vi "File_Writing_U6Instrumentation.vi"(8 "error in (no error)":errorcluster, 10 "Output":T1, 11 "Refnum in":refnum<k34>) -> (0 "error out":errorcluster, 3 "Refnum out":refnum<k34>)   [LabVIEW 2021]
uses:
  Control 1.ctl
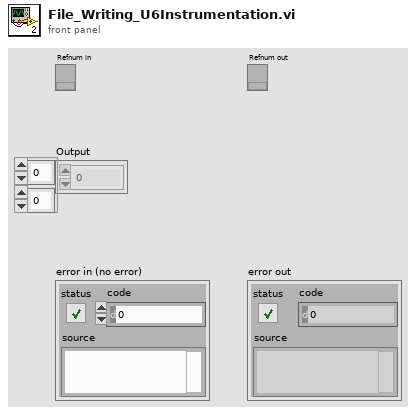
[diagram p1: front panel]
types:
  T1 = typedef "Control 1.ctl" = dbl[][]
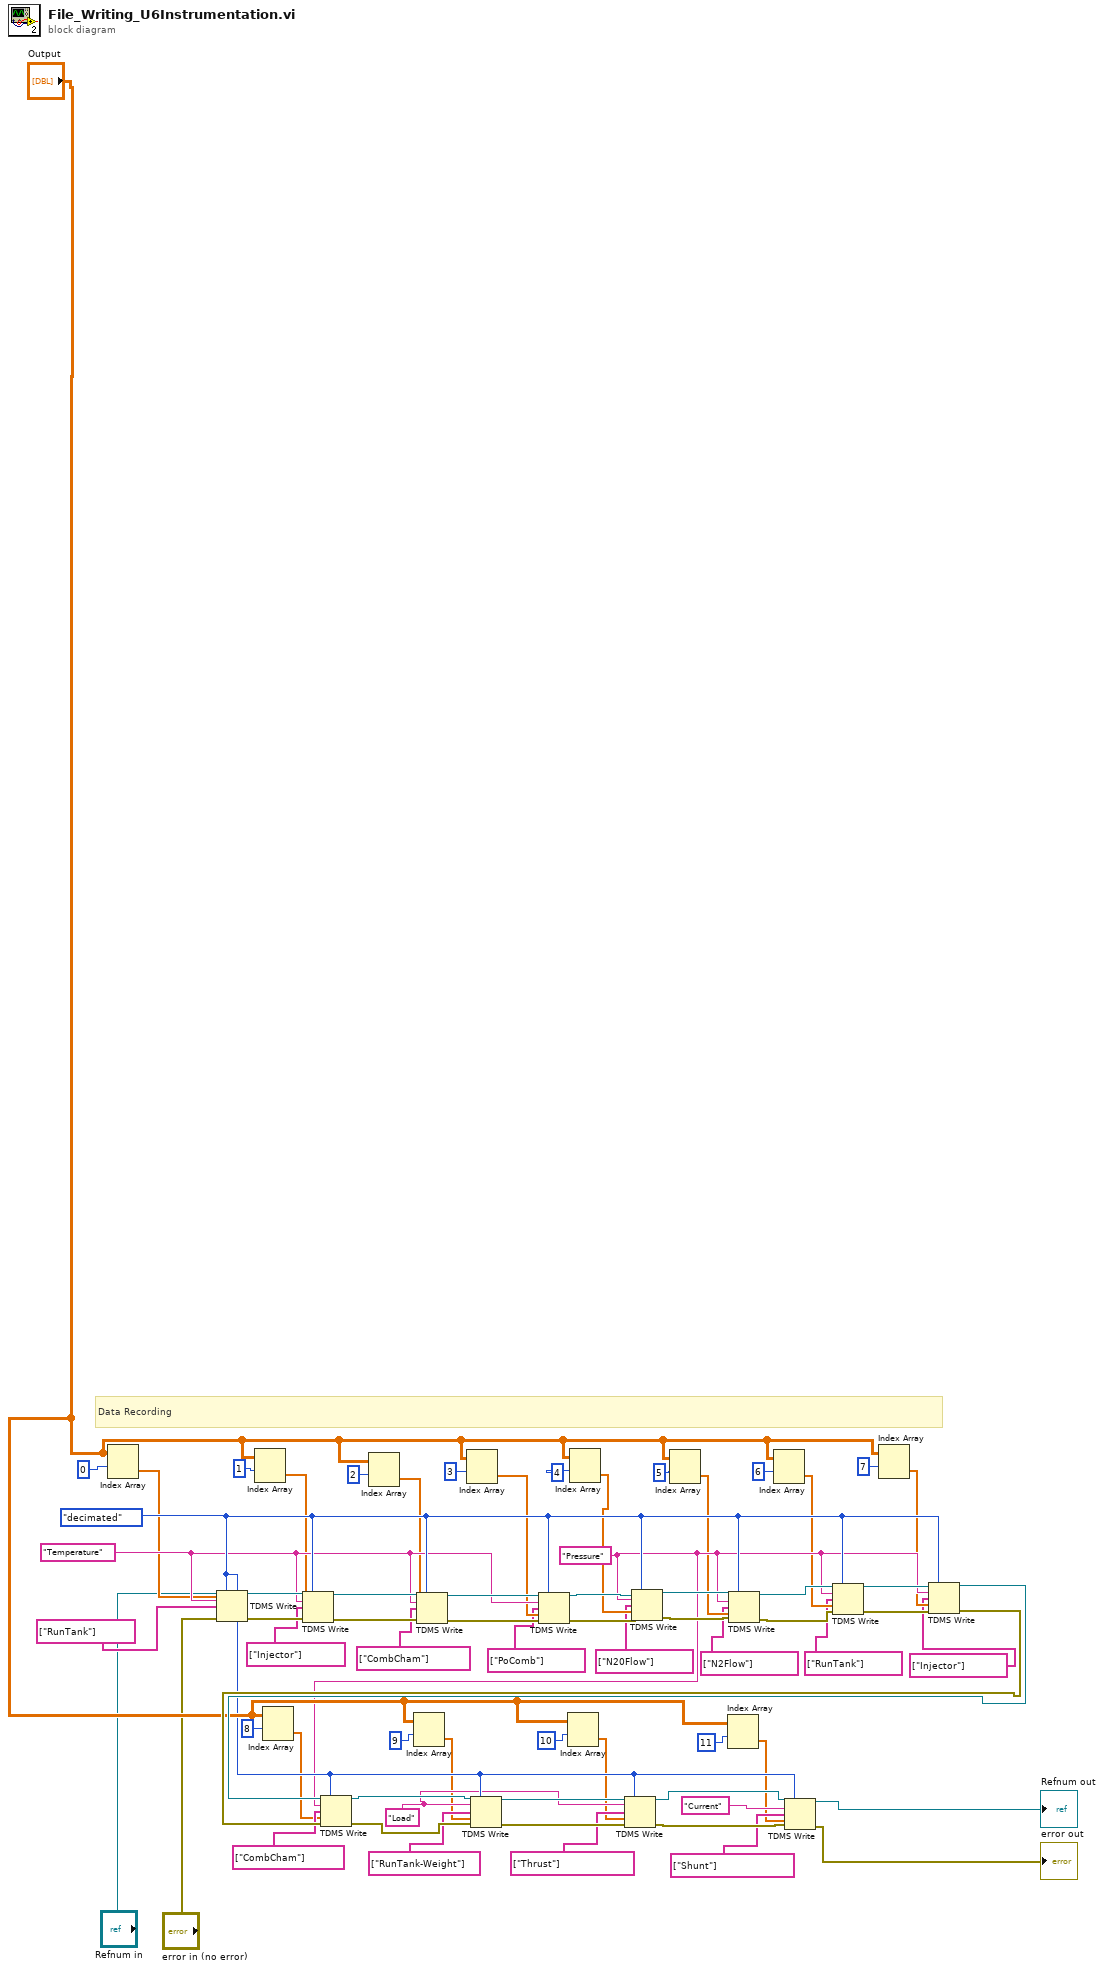
[diagram p0: block diagram]
diagram:
  w38 = "Load" ("group name in (Untitled)")
  w31 = "Pressure" ("group name in (Untitled)")
  w42 = enum16{"decimated", "interleaved"}."decimated" ("data layout (0:decimated)")
  w15 = "Temperature" ("group name in (Untitled)")
  # "Data Recording"
  n1 = Index Array(array="Output", index (row)=0) -> (element=w4:dbl[])  [unwired: 1 in]
  n2 = TDMS Write(0:"Refnum in", 1:w42, 5:w15, 7:string[] ["RunTank"] ("channel name(s) in (Untitled)"), 9:w4, 11:"error in (no error)") -> (4:w56:refnum<k34>, 15:w45:errorcluster)  [unwired: 2 out]
  n3 = Index Array(array="Output", index (row)=1) -> (element=w8:dbl[])  [unwired: 1 in]
  n4 = Index Array(array="Output", index (row)=8) -> (element=w28:dbl[])  [unwired: 1 in]
  n5 = TDMS Write(0:w56, 1:w42, 5:w15, 7:string[] ["Injector"] ("channel name(s) in (Untitled)"), 9:w8, 11:w45) -> (4:w57:refnum<k34>, 15:w46:errorcluster)  [unwired: 2 out]
  n6 = Index Array(array="Output", index (row)=2) -> (element=w10:dbl[])  [unwired: 1 in]
  n7 = Index Array(array="Output", index (row)=9) -> (element=w32:dbl[])  [unwired: 1 in]
  n8 = TDMS Write(0:w57, 1:w42, 5:w15, 7:string[] ["CombCham"] ("channel name(s) in (Untitled)"), 9:w10, 11:w46) -> (4:w58:refnum<k34>, 15:w47:errorcluster)  [unwired: 2 out]
  n9 = Index Array(array="Output", index (row)=3) -> (element=w13:dbl[])  [unwired: 1 in]
  n10 = TDMS Write(0:w58, 1:w42, 5:w15, 7:string[] ["PoComb"] ("channel name(s) in (Untitled)"), 9:w13, 11:w47) -> (4:w59:refnum<k34>, 15:w48:errorcluster)  [unwired: 2 out]
  n11 = Index Array(array="Output", index (row)=10) -> (element=w35:dbl[])  [unwired: 1 in]
  n12 = Index Array(array="Output", index (row)=4) -> (element=w17:dbl[])  [unwired: 1 in]
  n13 = TDMS Write(0:w59, 1:w42, 5:w31, 7:string[] ["N20Flow"] ("channel name(s) in (Untitled)"), 9:w17, 11:w48) -> (4:w60:refnum<k34>, 15:w49:errorcluster)  [unwired: 2 out]
  n14 = Index Array(array="Output", index (row)=5) -> (element=w20:dbl[])  [unwired: 1 in]
  n15 = Index Array(array="Output", index (row)=11) -> (element=w39:dbl[])  [unwired: 1 in]
  n16 = TDMS Write(0:w60, 1:w42, 5:w31, 7:string[] ["N2Flow"] ("channel name(s) in (Untitled)"), 9:w20, 11:w49) -> (4:w61:refnum<k34>, 15:w50:errorcluster)  [unwired: 2 out]
  n17 = Index Array(array="Output", index (row)=6) -> (element=w23:dbl[])  [unwired: 1 in]
  n18 = TDMS Write(0:w61, 1:w42, 5:w31, 7:string[] ["RunTank"] ("channel name(s) in (Untitled)"), 9:w23, 11:w50) -> (4:w62:refnum<k34>, 15:w51:errorcluster)  [unwired: 2 out]
  n19 = Index Array(array="Output", index (row)=7) -> (element=w26:dbl[])  [unwired: 1 in]
  n20 = TDMS Write(0:w62, 1:w42, 5:w31, 7:string[] ["Injector"] ("channel name(s) in (Untitled)"), 9:w26, 11:w51) -> (4:w63:refnum<k34>, 15:w52:errorcluster)  [unwired: 2 out]
  n21 = TDMS Write(0:w63, 1:w42, 5:w31, 7:string[] ["CombCham"] ("channel name(s) in (Untitled)"), 9:w28, 11:w52) -> (4:w64:refnum<k34>, 15:w53:errorcluster)  [unwired: 2 out]
  n22 = TDMS Write(0:w64, 1:w42, 5:w38, 7:string[] ["RunTank-Weight"] ("channel name(s) in (Untitled)"), 9:w32, 11:w53) -> (4:w65:refnum<k34>, 15:w54:errorcluster)  [unwired: 2 out]
  n23 = TDMS Write(0:w65, 1:w42, 5:w38, 7:string[] ["Thrust"] ("channel name(s) in (Untitled)"), 9:w35, 11:w54) -> (4:w66:refnum<k34>, 15:w55:errorcluster)  [unwired: 2 out]
  n24 = TDMS Write(0:w66, 1:w42, 5:"Current" ("group name in (Untitled)"), 7:string[] ["Shunt"] ("channel name(s) in (Untitled)"), 9:w39, 11:w55) -> (4:→"Refnum out":refnum<k34>, 15:→"error out":errorcluster)  [unwired: 2 out]
